vi "Multi Lockin.vi"(9 "Sig Index":i32=2, 10 "Ref Index":i32=1, 11 "array":waveform(dbl)[](array[waveform])) -> (0 "Active channel name":string, 1 "Ref channel name":string, 2 "Lock-in waveform output":waveform(dbl)[](array[waveform]), 3 "Lock-in output":T1 {"X" format="%#_3g"; "Y" format="%#_3g"; "R" format="%#_3g"}, 5 "Lock-in signals":waveform(dbl)[](graph)=[{"t0"=timestamp(3.0 s since 1904-01-01), "dt"=0.001, "Y"=array[1000 elements]}, {"t0"=timestamp(3649394049.416921 s since 1904-01-01), "dt"=0.001, "Y"=array[1000 elements], "attributes"=variant("NI_ChannelName"=variant(string "Dev1/ai0"), "NI_UnitDescription"=variant(string "Volts"))}])   [LabVIEW 2019]
doc: "This example demonstrates how to acquire a continuous amount of data (Waveform) using the DAQ device's internal clock. It also shows how to synchronize two devices for different device families (E Series, S Series, M Series, X Series, DSA, and SC Express), to simultaneously acquire the data.\n\nFor instructions on how to connect your signals to the DAQ device, refer to your device documentation."
uses:
  <vilib>/Waveform/WDTOps.llb/WDT Get Final Time Value DBL.vi
  <vilib>/Analysis/NI_AALPro.lvlib
panel:
  # "Lock-in"
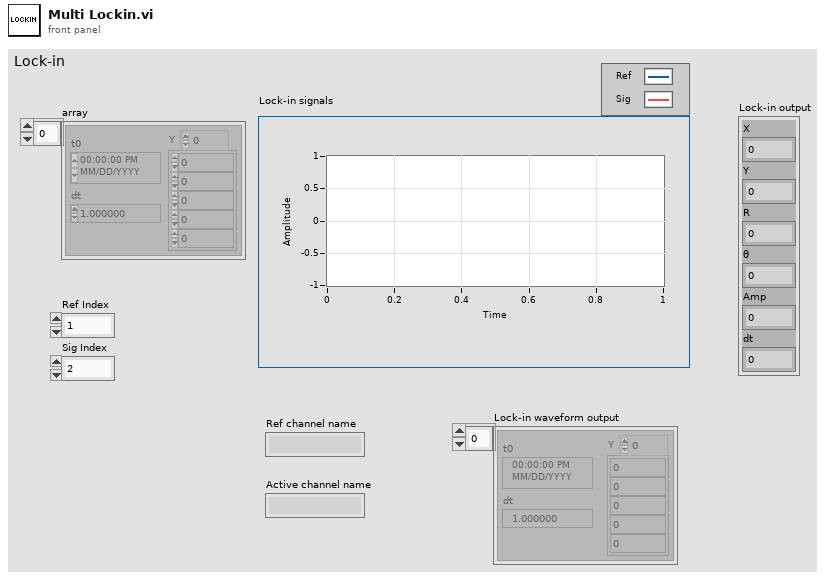
[diagram p1: front panel]
types:
  T1 = cluster{"X":dbl, "Y":dbl, "R":dbl, "θ":dbl, "Amp":dbl, "dt":dbl}
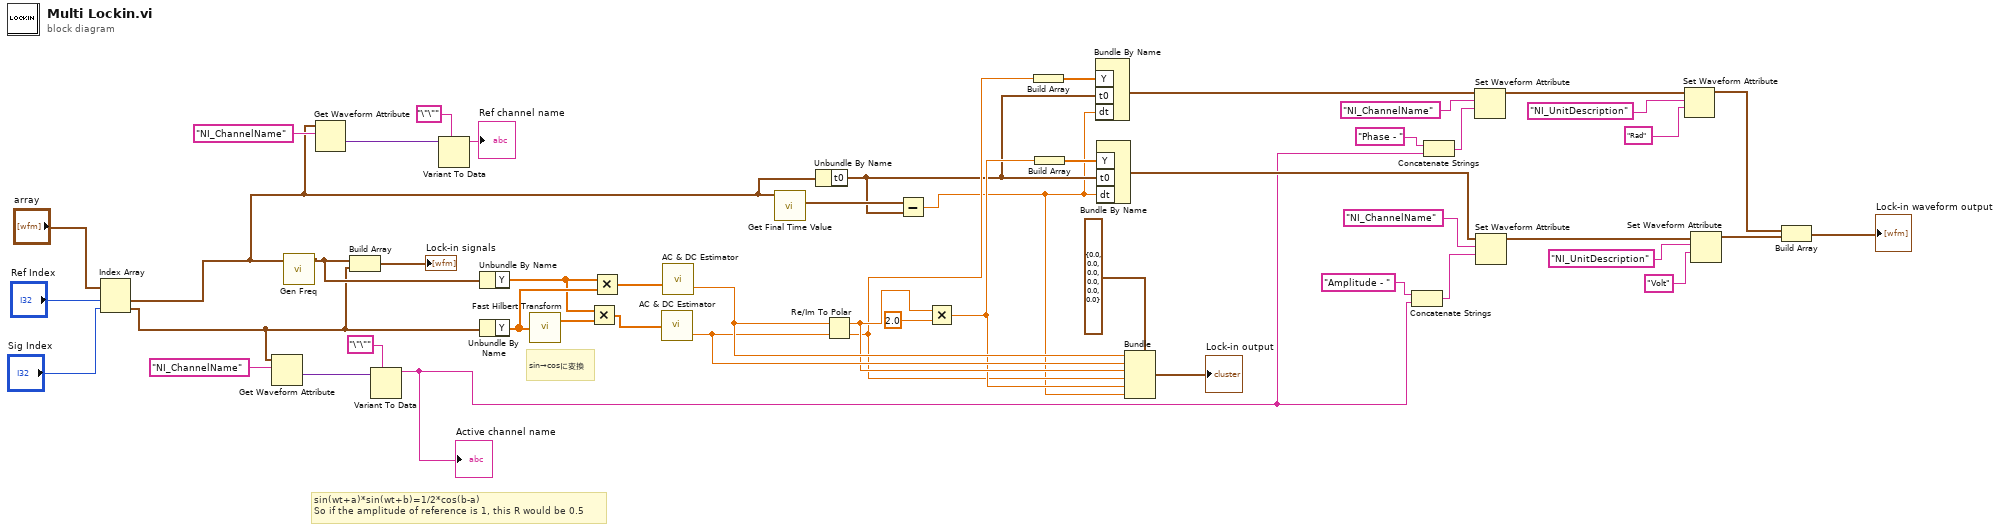
[diagram p0: block diagram]
diagram:
  # "sin(wt+a)*sin(wt+b)=1/2*cos(b-a)\nSo if the amplitude of reference is 1, this R would be 0.5"
  # "sin→cosに変換"
  n1 = Index Array(array="array", index #1="Ref Index", index #2="Sig Index") -> (element #1=w4:waveform(dbl), element #2=w11:waveform(dbl))
  n2 = Get Waveform Attribute(6:"NI_ChannelName" ("name"), 7:w11) -> (1:w9:variant)  [unwired: 2 in, 3 out]
  n3 = call "Gen Freq.vi"("Ref"=w4) -> ("Ref_PLL_Out"=w44:waveform(dbl))  [unwired: 10 in]
  n4 = Get Waveform Attribute(6:"NI_ChannelName" ("name"), 7:w4) -> (1:w2:variant)  [unwired: 2 in, 3 out]
  n5 = Build Array(w44, w11) -> (→"Lock-in signals":waveform(dbl)[])
  n6 = Variant To Data(type="\"\"" ("name"), Variant=w9) -> (data=w7:string)  [unwired: 1 in, 1 out]
  "Active channel name" <- w7
  n7 = Variant To Data(type="\"\"" ("name"), Variant=w2) -> (data=→"Ref channel name":string)  [unwired: 1 in, 1 out]
  n8 = Unbundle By Name(w44) -> ("Y"=w48:dbl[])
  n9 = Unbundle By Name(w11) -> ("Y"=w49:dbl[])
  n10 = call <vilib>:"Fast Hilbert Transform.vi"("X"=w49) -> ("Hilbert{X}"=w50:dbl[])  [unwired: 1 out]
  n11 = Multiply(x=w48, y=w50) -> (x*y=w46:dbl[])
  n12 = Multiply(x=w48, y=w49) -> (x*y=w47:dbl[])
  n13 = call <vilib>:"AC & DC Estimator.vi"("Signal (V)"=w46) -> ("DC estimate (V)"=w42:dbl)  [unwired: 1 out]
  n14 = call <vilib>:"AC & DC Estimator.vi"("Signal (V)"=w47) -> ("DC estimate (V)"=w43:dbl)  [unwired: 1 out]
  n15 = call-poly <vilib>:"Get Final Time Value.vi"("waveform in"=w4) -> ("tf"=w36:timestamp)  [unwired: 8 in, 2 out]
  n16 = Unbundle By Name(w4) -> ("t0"=w32:timestamp)
  n17 = Re/Im To Polar(2:w42, 3:w43) -> (0:w33:dbl, 1:w41:dbl)
  n18 = Subtract(x=w36, y=w32) -> (x-y=w6:dbl)
  n19 = Multiply(x=w41, y=2.0) -> (x*y=w38:dbl)
  n20 = Build Array(w33) -> (w34:dbl[])
  n21 = Build Array(w38) -> (w39:dbl[])
  n22 = Bundle By Name("Y"=w34, "t0"=w32, "dt"=w6) -> (w27:waveform(dbl))  [unwired: 1 in]
  n23 = Bundle By Name("Y"=w39, "t0"=w32, "dt"=w6) -> (w26:waveform(dbl))  [unwired: 1 in]
  n24 = Bundle(cluster=T1 {"X"=0.0, "Y"=0.0, "R"=0.0, "θ"=0.0, "Amp"=0.0, "dt"=0.0} ("input cluster"), "X"=w43, "Y"=w42, "R"=w41, "θ"=w33, "Amp"=w38, "dt"=w6) -> (→"Lock-in output":T1)
  n25 = Concatenate Strings("Amplitude - " ("name"), w7) -> (w21:string)
  n26 = Concatenate Strings("Phase - " ("name"), w7) -> (w22:string)
  n27 = Set Waveform Attribute(5:w22, 6:"NI_ChannelName" ("name"), 7:w27) -> (3:w17:waveform(dbl))  [unwired: 1 in, 2 out]
  n28 = Set Waveform Attribute(5:w21, 6:"NI_ChannelName" ("name"), 7:w26) -> (3:w15:waveform(dbl))  [unwired: 1 in, 2 out]
  n29 = Set Waveform Attribute(5:"Rad" ("name"), 6:"NI_UnitDescription" ("name"), 7:w17) -> (3:w16:waveform(dbl))  [unwired: 1 in, 2 out]
  n30 = Set Waveform Attribute(5:"Volt" ("name"), 6:"NI_UnitDescription" ("name"), 7:w15) -> (3:w14:waveform(dbl))  [unwired: 1 in, 2 out]
  n31 = Build Array(w16, w14) -> (→"Lock-in waveform output":waveform(dbl)[])
